vi "img test7(track).vi"() -> ()   [LabVIEW 2009]
uses:
  <vilib>/vision/NI_Vision_Development_Module.lvlib
panel:
  out "positions":dbl[][](array[numeric])
  in  "playing?":bool
  out "XY Graph":cluster{"Numeric":dbl, "Numeric":dbl}[](graph)
  in  "frame jump":i32=3
  out "Array":dbl[][](array[numeric])
  out "Image 4":T1(plugin-control)
  in  "milliseconds to wait":u32=200
  in  "start":i32
  out "Image 5":T1(plugin-control)
  out "Image 3":T1(plugin-control)
  in  "Range":cluster{"Lower value":sgl, "Upper value":sgl}={"Lower value"=30.0, "Upper value"=90.0} {"Upper value" format="%.2f"; "Lower value" format="%.2f"}
  out "Image 2":T1(plugin-control)
  in  "AVI Path":path=path "C:/Users/Kokum Weeratunga/Desktop/img processing/ChongWei vs LinDan (japan open 2010).avi"
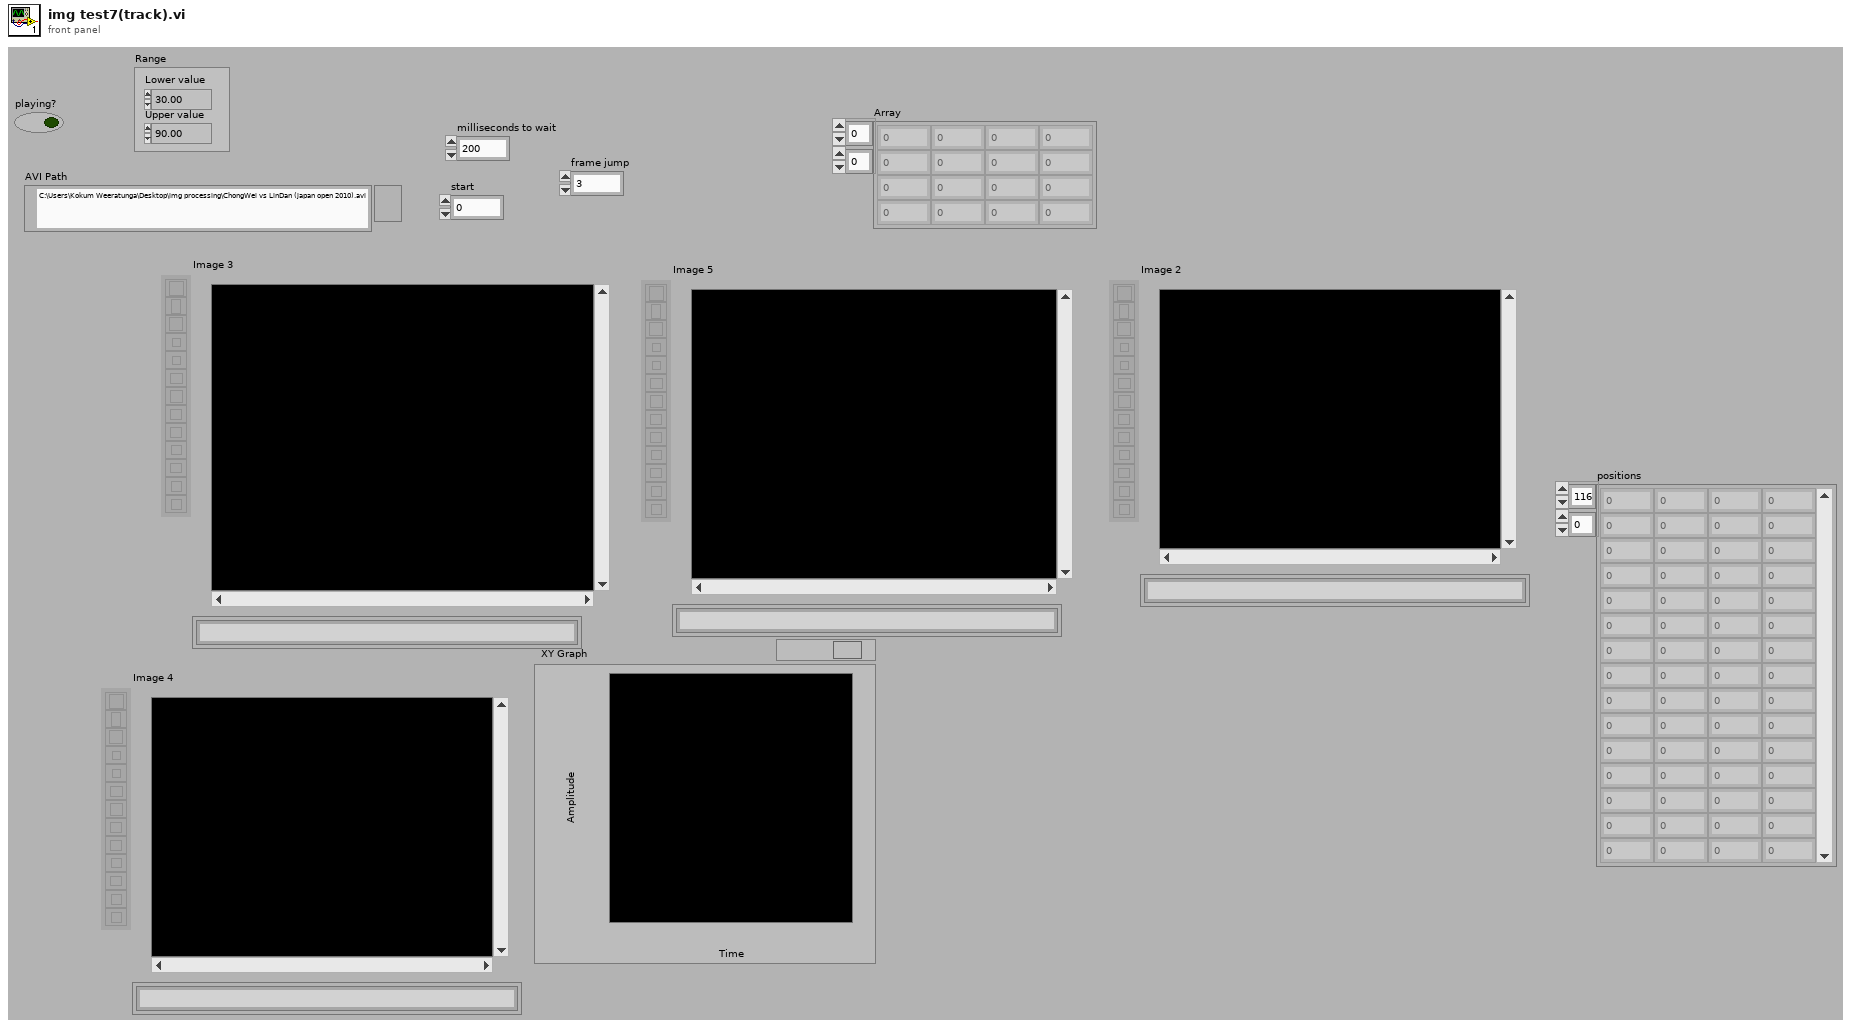
[diagram p1: front panel]
types:
  T1 = typedef "IMAQ Image.ctl" = refnum<image>
  T2 = typedef "Image Type" = u32
  T3 = typedef "AviRefnum.ctl" = refnum<k1>
  T4 = enum32{"AutoM", "Close", "Dilate", "Erode", "Gradient", "Gradient out", "Gradient in", "Hit miss", "Open", "PClose", "POpen", "Thick", "Thin"}
  T5 = enum32{"AutoM", "Close", "Dilate", "Erode", "Gradient", "Gradient in", "Gradient out", "HitMiss", "Open", "PClose", "POpen", "Thick", "Thin"}
  T6 = typedef "Particle Parameters" = i32
  T7 = cluster{"Numeric":dbl, "Numeric":dbl, "Numeric":dbl, "Numeric":dbl}
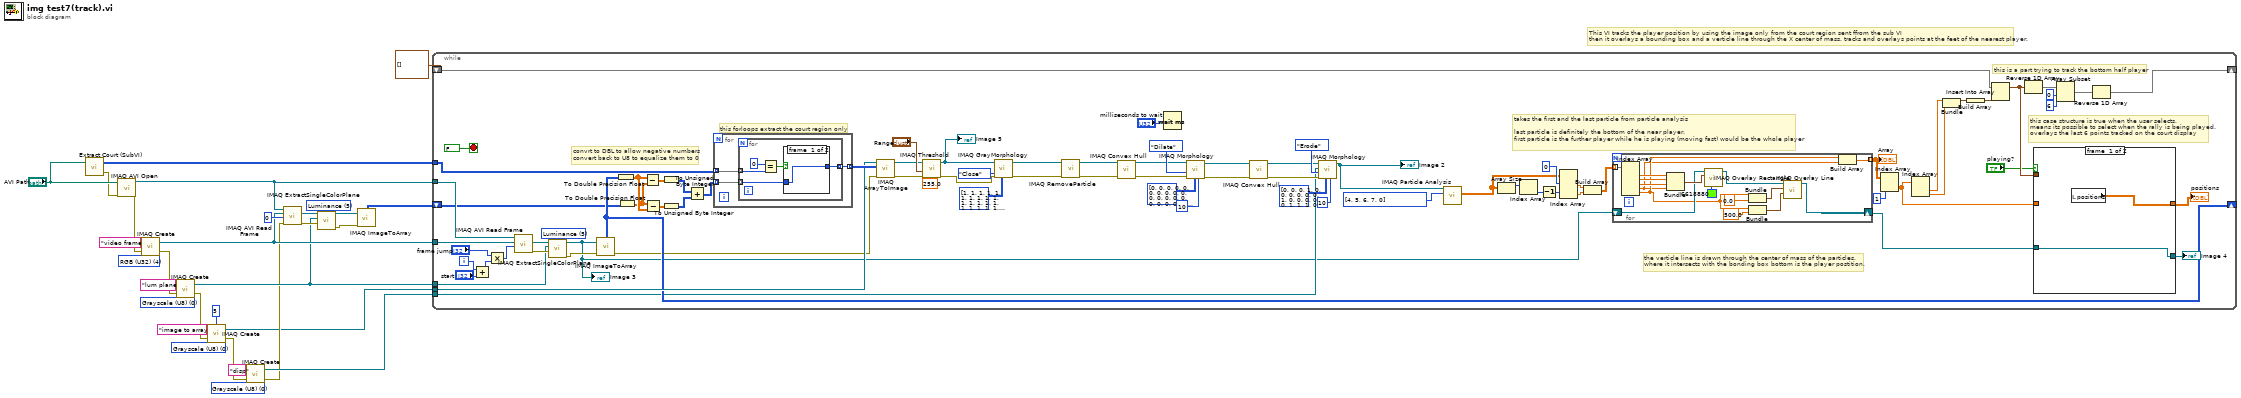
[diagram p0: block diagram]
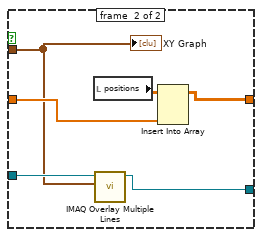
[diagram p2: hidden frame]
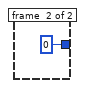
[diagram p3: hidden frame]
diagram:
  w13 = T2 0 items=["Grayscale (U8)", "Grayscale (I16)", "Grayscale (SGL)", "Complex (CSG)", "RGB (U32)", "HSL (U32)", "RGB (U64)", "Grayscale (U16)"] ("Image Type")
  w21 = 5 items=["Red", "Green", "Blue", "Hue", "Saturation", "Luminance", "Value", "Intensity"] ("Color Plane")
  w23 = T2 0 items=["Grayscale (U8)", "Grayscale (I16)", "Grayscale (SGL)", "Complex (CSG)", "RGB (U32)", "HSL (U32)", "RGB (U64)", "Grayscale (U16)"] ("Image Type")
  w27 = T2 0 items=["Grayscale (U8)", "Grayscale (I16)", "Grayscale (SGL)", "Complex (CSG)", "RGB (U32)", "HSL (U32)", "RGB (U64)", "Grayscale (U16)"] ("Image Type")
  w25 = T2 4 items=["Grayscale (U8)", "Grayscale (I16)", "Grayscale (SGL)", "Complex (CSG)", "RGB (U32)", "HSL (U32)", "RGB (U64)", "Grayscale (U16)"] ("Image Type")
  # "This VI tracks the player position by using the image only from the court region sent ffrom the sub VI\nthen it overlays a bounding box and a verticle line through the X center of mass. tracks and overlays points at the feet of the nearest player."
  n1 = call "Extract Court (SubVI).vi"("AVI Path"="AVI Path") -> ("error out"=w29:errorcluster, "Court pixels out"=w3:u8[][])  [unwired: 1 in]
  n2 = call "IMAQ AVI Open"("error in (no error)"=w29, "AVI Path"="AVI Path") -> ("error out"=w9:errorcluster, "Avi Refnum"=w19:T3)  [unwired: 8 in]
  n3 = call "IMAQ Create"("Image Name"="video frame", "Image Type"=w25, "error in (no error)"=w9) -> ("New Image"=w17:T1, "error out"=w8:errorcluster)  [unwired: 2 in]
  n4 = call "IMAQ Create"("Image Name"="lum plane", "Image Type"=w27, "error in (no error)"=w8) -> ("New Image"=w16:T1, "error out"=w7:errorcluster)  [unwired: 2 in]
  n5 = call "IMAQ Create"("Border Size"=5, "Image Name"="image to array", "Image Type"=w23, "error in (no error)"=w7) -> ("New Image"=w2:T1, "error out"=w6:errorcluster)  [unwired: 1 in]
  n6 = call "IMAQ Create"("Image Name"="disp", "Image Type"=w13, "error in (no error)"=w6) -> ("New Image"=w11:T1, "error out"=w5:errorcluster)  [unwired: 2 in]
  n7 = call "IMAQ AVI Read Frame"("error in (no error)"=w5, "Frame Number"=u32 0, "Image"=w17, "Avi Refnum"=w19) -> ("error out"=w20:errorcluster, "Image Out"=w22:T1)  [unwired: 4 in, 2 out]
  n8 = call "IMAQ ExtractSingleColorPlane"("Color Plane"=w21, "error in (no error)"=w20, "Image Dst"=w16, "Image Src"=w22) -> ("error out"=w10:errorcluster, "Image Dst Out"=w14:T1)  [unwired: 6 in]
  n9 = call "IMAQ ImageToArray"("error in (no error)"=w10, "Image"=w14) -> ("Image Pixels (U8)"=w15:u8[][])  [unwired: 2 in, 4 out]
  n10 = while {
    tunnel: w19 -> [w109]
    tunnel: w17 -> [w59]
    tunnel: w3 -> [w108]
    tunnel: w16 -> [w61]
    tunnel: w2 -> [w101]
    shift-right: [w100] -> _
    shift-left: w15 -> [w99]
    tunnel: w11 -> [w63]
    shift-right: [w41] -> _
    shift-left: cluster{"Numeric":dbl, "Numeric":dbl}[] [] -> [w47]
    i -> [w92]
    stop <- FALSE stop-if-true
    w62 = T6[] [4, 5, 6, 7, 0] items=["Center of Mass X", "Center of Mass Y", "First Pixel X", "First Pixel Y", "Bounding Rect Left", "Bounding Rect Top", "Bounding Rect Right", "Bounding Rect Bottom", "Max Feret Diameter Start X", "Max Feret Diameter Start Y", "Max Feret Diameter End X", "Max Feret Diameter End Y", "Max Horiz. Segment Length Left", "Max Horiz. Segment Length Right", "Max Horiz. Segment Length Row", "-", "Bounding Rect Width", "Bounding Rect Height", "Bounding Rect Diagonal", "Perimeter", "Convex Hull Perimeter", "Holes' Perimeter", "Max Feret Diameter", "Equivalent Ellipse Major Axis", "Equivalent Ellipse Minor Axis", "Equivalent Ellipse Minor Axis (Feret)", "Equivalent Rect Long Side", "Equivalent Rect Short Side", "Equivalent Rect Diagonal", "Equivalent Rect Short Side (Feret)", "Average Horiz. Segment Length", "Average Vert. Segment Length", "Hydraulic Radius", "Waddel Disk Diameter", "-", "Area", "Holes' Area", "Particle & Holes' Area", "Convex Hull Area", "Image Area", "-", "Number of Holes", "Number of Horiz. Segments", "Number of Vert. Segments", "-", "Orientation", "Max Feret Diameter Orientation", "-", "% Area/Image Area", "% Area/(Particle & Holes' Area)", "Ratio of Equivalent Ellipse Axes", "Ratio of Equivalent Rect Sides", "-", "Elongation Factor", "Compactness Factor", "Heywood Circularity Factor", "Type Factor", "-", "Sum X", "Sum Y", "Sum XX", "Sum XY", "Sum YY", "Sum XXX", "Sum XXY", "Sum XYY", "Sum YYY", "-", "Moment of Inertia XX", "Moment of Inertia XY", "Moment of Inertia YY", "Moment of Inertia XXX", "Moment of Inertia XXY", "Moment of Inertia XYY", "Moment of Inertia YYY", "Norm. Moment of Inertia XX", "Norm. Moment of Inertia XY", "Norm. Moment of Inertia YY", "Norm. Moment of Inertia XXX", "Norm. Moment of Inertia XXY", "Norm. Moment of Inertia XYY", "Norm. Moment of Inertia YYY", "Hu Moment 1", "Hu Moment 2", "Hu Moment 3", "Hu Moment 4", "Hu Moment 5", "Hu Moment 6", "Hu Moment 7"] ("Pixel Measurements")
    w110 = 5 items=["Red", "Green", "Blue", "Hue", "Saturation", "Luminance", "Value", "Intensity"] ("Color Plane")
    # "this case structure is true when the user selects. \nmeans its possible to select when the rally is being played.\noverlays the last 6 points tracked on the court display"
    # "this is a part trying to track the bottom half player"
    # "the verticle line is drawn through the center of mass of the particles. \nwhere it intersects with the bonding box bottom is the player postition."
    # "takes the first and the last particle from particle analysis\n\nlast particle is definitely the bottom of the near player. \nfirst particle is the further player while he is playing (moving fast) would be the whole player"
    # "convrt to DBL to allow negative numbers\nconvert back to U8 to equalize them to 0"
    # "this forloops extract the court region only"
    n11 = Add(x=w92, y="start") -> (x+y=w91:i32)
    n12 = Multiply(x="frame jump", y=w91) -> (x*y=w105:i32)
    n13 = call "IMAQ AVI Read Frame"("Frame Number"=w105, "Image"=w59, "Avi Refnum"=w109) -> ("error out"=w111:errorcluster, "Image Out"=w60:T1)  [unwired: 5 in, 2 out]
    n14 = call "IMAQ ExtractSingleColorPlane"("Color Plane"=w110, "error in (no error)"=w111, "Image Dst"=w61, "Image Src"=w60) -> ("error out"=w85:errorcluster, "Image Dst Out"=w58:T1)  [unwired: 6 in]
    "Image 3" <- w58
    n15 = call "IMAQ ImageToArray"("error in (no error)"=w85, "Image"=w58) -> ("error out"=w84:errorcluster, "Image Pixels (U8)"=w100:u8[][])  [unwired: 2 in, 3 out]
    n16 = To Double Precision Float(number=w100) -> (double precision float=w89:dbl[][])
    n17 = To Double Precision Float(number=w99) -> (double precision float=w88:dbl[][])
    n18 = Subtract(x=w89, y=w88) -> (x-y=w87:dbl[][])
    n19 = Subtract(x=w88, y=w89) -> (x-y=w86:dbl[][])
    n20 = To Unsigned Byte Integer(number=w87) -> (unsigned 8bit integer=w98:u8[][])
    n21 = To Unsigned Byte Integer(number=w86) -> (unsigned 8bit integer=w97:u8[][])
    n22 = Add(x=w98, y=w97) -> (x+y=w96:u8[][])
    n23 = for {
      tunnel: w108 -> [w138] mode=indexing
      tunnel: [w137] -> w106 mode=indexing
      tunnel: w96 -> [w136] mode=indexing
      n24 = for {
        tunnel: w138 -> [w143] mode=indexing
        tunnel: [w140] -> w137 mode=indexing
        tunnel: w136 -> [w139] mode=indexing
        n25 = Equal?(x=u8 0, y=w143) -> (x = y?=w141:bool)
        n26 = case shown="True" w141 {
          tunnel: [w144 u8 0 ("x")] -> w140
          tunnel: w139 -> [w144 _]
          frame #0 {
          }
          frame #1 {
          }
        }
      }
    }
    n27 = call "IMAQ ArrayToImage"("error in (no error)"=w84, "Image Pixels (U8)"=w106, "Image"=w101) -> ("error out"=w83:errorcluster, "Image Out"=w65:T1)  [unwired: 7 in]
    n28 = call "IMAQ Threshold"("Replace Value"=sgl 255.0, "error in (no error)"=w83, "Range"="Range", "Image Src"=w65) -> ("error out"=w82:errorcluster, "Image Dst Out"=w95:T1)  [unwired: 6 in]
    "Image 5" <- w95
    n29 = call "IMAQ GrayMorphology"("Structuring Element"=i32[][] [[1, 1, 1, 1, 1, 1, 1, 1, 1], [1, 1, 1, 1, 1, 1, 1, 1, 1], [1, 1, 1, 1, 1, 1, 1, 1, 1], [1, 1, 1, 1, 1, 1, 1, 1, 1], [1, 1, 1, 1, 1, 1, 1, 1, 1], [1, 1, 1, 1, 1, 1, 1, 1, 1], [1, 1, 1, 1, 1, 1, 1, 1, 1], [1, 1, 1, 1, 1, 1, 1, 1, 1], [1, 1, 1, 1, 1, 1, 1, 1, 1]], "error in (no error)"=w82, "Operation"=T5."Close", "Image Src"=w95) -> ("error out"=w80:errorcluster, "Image Dst Out"=w81:T1)  [unwired: 6 in]
    n30 = call "IMAQ RemoveParticle"("error in (no error)"=w80, "Image Src"=w81) -> ("error out"=w79:errorcluster, "Image Dst Out"=w78:T1)  [unwired: 8 in]
    n31 = call "IMAQ Convex Hull"("error in (no error)"=w79, "Image Src"=w78) -> ("error out"=w74:errorcluster, "Image Dst Out"=w64:T1)  [unwired: 8 in]
    n32 = Wait (ms)(milliseconds to wait="milliseconds to wait") -> ()  [unwired: 1 out]
    n33 = call "IMAQ Morphology"("Number of iterations (1)"=10, "Structuring Element"=i32[][] [[0, 0, 0, 0, 0, 0, 0], [0, 0, 0, 0, 0, 0, 0], [0, 0, 0, 0, 0, 0, 0], [0, 0, 0, 0, 0, 0, 0], [0, 0, 1, 1, 1, 0, 0], [0, 0, 0, 1, 0, 0, 0], [0, 0, 0, 1, 0, 0, 0]], "error in (no error)"=w74, "Operation"=T4."Dilate", "Image Src"=w64) -> ("error out"=w68:errorcluster, "Image Dst Out"=w69:T1)  [unwired: 5 in]
    n34 = call "IMAQ Convex Hull"("error in (no error)"=w68, "Image Src"=w69) -> ("error out"=w66:errorcluster, "Image Dst Out"=w67:T1)  [unwired: 8 in]
    n35 = call "IMAQ Morphology"("Number of iterations (1)"=10, "Structuring Element"=i32[][] [[0, 0, 0, 1, 0, 0, 0], [0, 0, 0, 1, 0, 0, 0], [0, 0, 1, 1, 1, 0, 0], [0, 0, 0, 0, 0, 0, 0], [0, 0, 0, 0, 0, 0, 0], [0, 0, 0, 0, 0, 0, 0], [0, 0, 0, 0, 0, 0, 0]], "error in (no error)"=w66, "Operation"=T4."Erode", "Image Dst"=w63, "Image Src"=w67) -> ("Image Dst Out"=w49:T1)  [unwired: 4 in, 1 out]
    "Image 2" <- w49
    n36 = call "IMAQ Particle Analysis"("Pixel Measurements"=w62, "Image"=w49) -> ("Particle Measurements (Pixels)"=w51:dbl[][])  [unwired: 4 in, 5 out]
    n37 = Array Size(array=w51) -> (size(s)=w57:i32[])
    n38 = Index Array(array=w57) -> (element=w54:i32)  [unwired: 1 in]
    n39 = Decrement(x=w54) -> (x-1=w55:i32)
    n40 = Index Array(array=w51, index (row) #1=0 ("index (row)"), index (row) #2=w55) -> (element #1=w53:dbl[], element #2=w52:dbl[])  [unwired: 2 in]
    n41 = Build Array(w53, w52) -> (w50:dbl[][])
    n42 = for {
      shift-right: [w125] -> w32
      shift-left: w58 -> [w131]
      tunnel: w50 -> [w129] mode=indexing
      tunnel: [w122] -> w48 mode=indexing
      n43 = Index Array(array=w129) -> (element #1=w135:dbl, element #2=w134:dbl, element #3=w133:dbl, element #4=w120:dbl, element #5=w121:dbl)  [unwired: 5 in]
      n44 = Bundle("Numeric"=w135, "Numeric"=w134, "Numeric"=w133, "Numeric"=w120) -> (w132:T7)  [unwired: 1 in]
      n45 = call "IMAQ Overlay Rectangle"("Color"=u32 6618880, "Rectangle"=w132, "Image"=w131) -> ("Image Out"=w128:T1)  [unwired: 7 in, 1 out]
      n46 = Bundle("Numeric"=w121, "element"=500.0) -> (w124:cluster{"Numeric":dbl, "element":dbl})  [unwired: 1 in]
      n47 = Bundle("Numeric"=w121, "element"=0.0) -> (w126:cluster{"Numeric":dbl, "element":dbl})  [unwired: 1 in]
      n48 = call "IMAQ Overlay Line"("End Point"=w124, "Start Point"=w126, "Image"=w128) -> ("Image Out"=w125:T1)  [unwired: 7 in, 1 out]
      n49 = Build Array(w121, w120) -> (w122:dbl[])
    }
    "Array" <- w48
    n50 = Index Array(array=w48, index (row)=1) -> (element=w38:dbl[])  [unwired: 1 in]
    n51 = Index Array(array=w38) -> (element #1=w36:dbl, element #2=w35:dbl)  [unwired: 2 in]
    n52 = Bundle("Numeric"=w36, "Numeric"=w35) -> (w34:cluster{"Numeric":dbl, "Numeric":dbl})  [unwired: 1 in]
    n53 = Build Array(w34) -> (w33:cluster{"Numeric":dbl, "Numeric":dbl}[])
    n54 = Insert Into Array(array=w47, new element=w33) -> (w42:cluster{"Numeric":dbl, "Numeric":dbl}[])  [unwired: 1 in]
    n55 = Reverse 1D Array(array=w42) -> (reversed array=w46:cluster{"Numeric":dbl, "Numeric":dbl}[])
    n56 = case shown="True" "playing?" {
      tunnel: w42 -> [_ w114]
      tunnel: w38 -> [_ w118]
      tunnel: [w113 w119] -> w37
      tunnel: w32 -> [w112 w116]
      tunnel: [w112 w115] -> w31
      frame #0 {
        n57 = local read "positions"() -> (w113:dbl[][])
      }
      frame #1 {
        n58 = local read "positions"() -> (w117:dbl[][])
        n59 = call "IMAQ Overlay Multiple Lines"("Line End Points"=w114, "Image"=w116) -> ("Image Out"=w115:T1)  [unwired: 8 in, 1 out]
        n60 = Insert Into Array(array=w117, new element=w118) -> (w119:dbl[][])  [unwired: 2 in]
        "XY Graph" <- w114
      }
    }
    "Image 4" <- w31
    "positions" <- w37
    n61 = Array Subset(array=w46, index=0, length=6) -> (w43:cluster{"Numeric":dbl, "Numeric":dbl}[])
    n62 = Reverse 1D Array(array=w43) -> (reversed array=w41:cluster{"Numeric":dbl, "Numeric":dbl}[])
  }
